vi "Pic Overlay c Point.vi"(8 "error in (no error)":errorcluster, 11 "LF2R IDE in":refnum<class "Main Panel.lvclass">) -> (0 "error out":errorcluster, 3 "LF2R IDE out":refnum<class "Main Panel.lvclass">)   [LabVIEW 2018, in "Main Panel.lvlib" / "Main Panel.lvclass"]
uses:
  Main Panel.lvclass
  Main Panel.lvclass/Main Panel.ctl
  Picture Process/Picture Process.lvclass
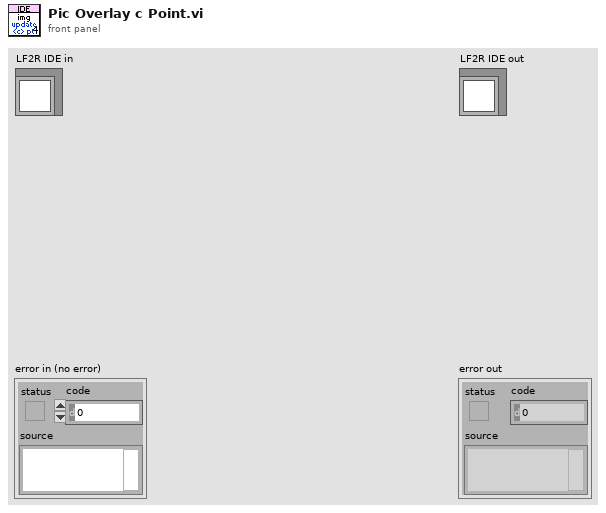
[diagram p1: front panel]
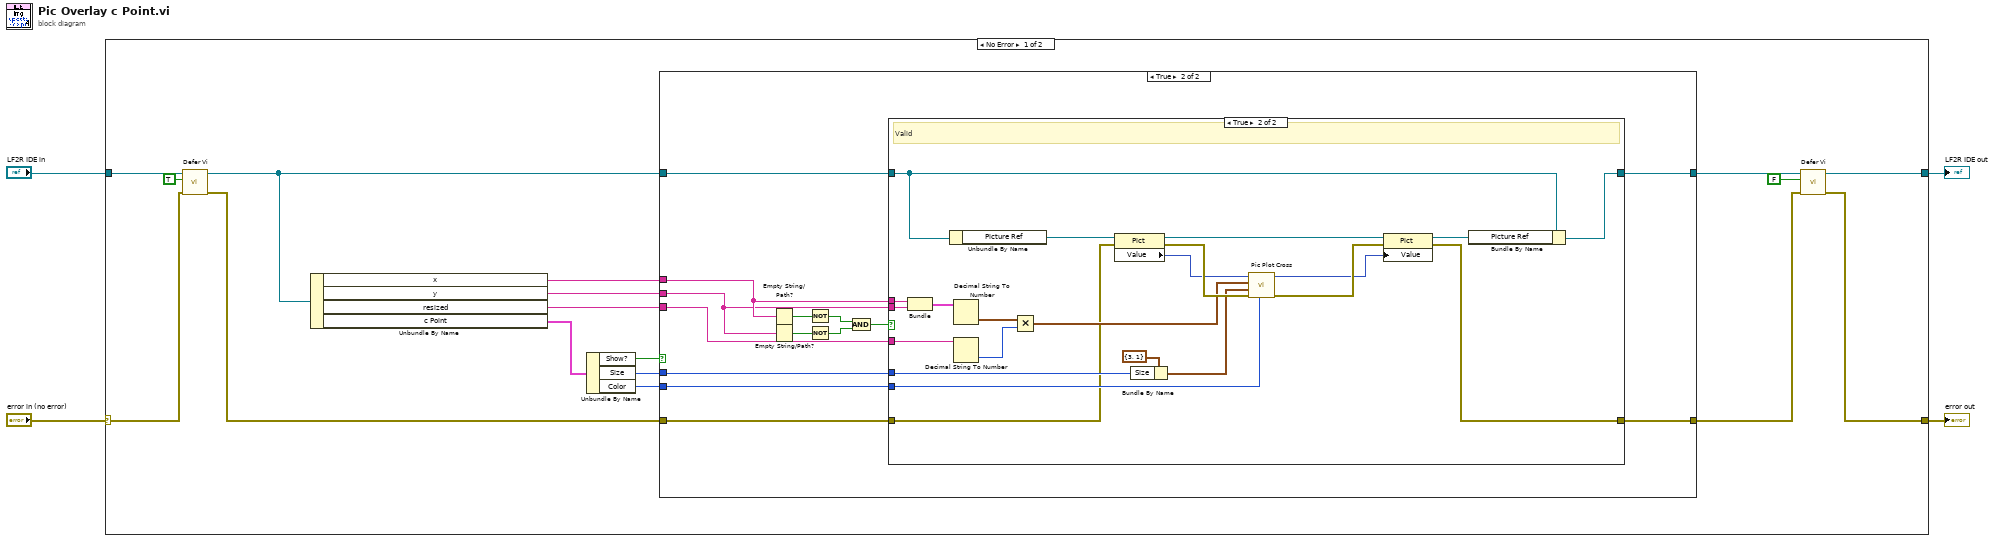
[diagram p0: block diagram]
diagram:
  n1 = case shown="No Error" "error in (no error)" {
    selector: "error in (no error)" -> [w12 w63]
    tunnel: [w6 w63] -> w3
    tunnel: [w8 w62] -> w1
    tunnel: "LF2R IDE in" -> [w14 w62]
    frame No Error {
      n2 = call "Defer Vi.vi"("error in (no error)"=w12, "Defer Updates?"=TRUE, "Main Panel in"=w14) -> ("error out"=w11:errorcluster, "Main Panel out"=w13:refnum<class "Main Panel.lvclass">)  [unwired: 7 in]
      n3 = Unbundle By Name(w13) -> ("x"=w20:string, "y"=w19:string, "resized"=w21:string, "c Point"=w18:cluster{"Size":i32, "Color":u32, "Show?":bool})
      n4 = Unbundle By Name(w18) -> ("Show?"=w17:bool, "Size"=w16:i32, "Color"=w15:u32)
      n5 = case shown="True" w17 {
        tunnel: w13 -> [w23 w37]
        tunnel: [w22 w36] -> w7
        tunnel: w21 -> [_ w35]
        tunnel: w11 -> [w22 w34]
        tunnel: w20 -> [_ w33]
        tunnel: w19 -> [_ w32]
        tunnel: [w23 w26] -> w9
        tunnel: w16 -> [_ w25]
        tunnel: w15 -> [_ w24]
        frame False {
        }
        frame True {
          n6 = Empty String/Path?(string/path=w33) -> (empty?=w31:bool)
          n7 = Empty String/Path?(string/path=w32) -> (empty?=w30:bool)
          n8 = Not(x=w31) -> (.not. x?=w29:bool)
          n9 = Not(x=w30) -> (.not. x?=w28:bool)
          n10 = And(x=w29, y=w28) -> (x .and. y?=w27:bool)
          n11 = case shown="True" w27 {
            tunnel: w37 -> [w39 w55]
            tunnel: [w38 w42] -> w36
            tunnel: w35 -> [_ w61]
            tunnel: w34 -> [w38 w43]
            tunnel: w33 -> [_ w58]
            tunnel: w32 -> [_ w57]
            tunnel: [w39 w41] -> w26
            tunnel: w25 -> [_ w46]
            tunnel: w24 -> [_ w44]
            frame False {
              # "Invalid"
            }
            frame True {
              # "Valid"
              n12 = Bundle("x"=w58, "y"=w57) -> (w56:cluster{"x":string, "y":string})  [unwired: 1 in]
              n13 = Unbundle By Name(w55) -> ("Picture Ref"=w54:refnum<vi>)
              n14 = Decimal String To Number(string=w56) -> (number=w60:cluster{"x":i32, "y":i32})  [unwired: 2 in, 1 out]
              n15 = Decimal String To Number(string=w61) -> (number=w59:i32)  [unwired: 2 in, 1 out]
              n16 = Multiply(x=w60, y=w59) -> (x*y=w48:cluster{"x":i32, "y":i32})
              n17 = property class="Pict"(reference=w54, error in=w43) -> (reference out=w53:refnum<vi>, error out=w52:errorcluster, "Value"=w49:picture)
              n18 = Bundle By Name(cluster=cluster{"Size":i32, "Width":u16} {"Size"=3, "Width"=1} ("Line"), "Size"=w46) -> (w45:cluster{"Size":i32, "Width":u16})
              n19 = call "Pic Plot Cross.vi"("Color"=w44, "error in (no error)"=w52, "Line"=w45, "Position"=w48, "Picture in"=w49) -> ("error out"=w51:errorcluster, "Picture out"=w50:picture)  [unwired: 5 in]
              n20 = property class="Pict"(reference=w53, error in=w51, "Value"=w50) -> (reference out=w40:refnum<vi>, error out=w42:errorcluster)
              n21 = Bundle By Name(cluster=w55, "Picture Ref"=w40) -> (w41:refnum<class "Main Panel.lvclass">)
            }
          }
        }
      }
      n22 = call "Defer Vi.vi"("error in (no error)"=w7, "Defer Updates?"=FALSE, "Main Panel in"=w9) -> ("error out"=w6:errorcluster, "Main Panel out"=w8:refnum<class "Main Panel.lvclass">)  [unwired: 7 in]
    }
    frame Error {
    }
  }
  "error out" <- w3
  "LF2R IDE out" <- w1
